vi "Finish.vi"   [LabVIEW 2017]
doc: "This VI is called just before exiting. It is expected to close I/O refnum, save collected data, etc."
types:
  T1 = typedef "WPI_JoystickDevRef.ctl" = cluster{"Device":T2}
  T2 = typedef "WPI_JoystickDeviceEnum.ctl" = enum16{"USB 0", "USB 1", "USB 2", "USB 3", "USB 4", "USB 5"}
  T3 = typedef "WPI_SolenoidDevRef.ctl" = cluster{"DevStatus":errorcluster, "Pneumatics Control Module":u8, "Forward Solenoid Channel":T4, "Reverse Solenoid Channel":T4}
  T4 = typedef "WPI_SolenoidChannel.ctl" = enum8{"Solenoid 0", "Solenoid 1", "Solenoid 2", "Solenoid 3", "Solenoid 4", "Solenoid 5", "Solenoid 6", "Solenoid 7", "Invalid"}
  T5 = typedef "WPI_EncoderDevRef.ctl" = cluster{"DevStatus":errorcluster, "EncoderIndex":T6, "CounterIndex":T7, "DistancePerCount":dbl, "Decoding Type":T8}
  T6 = typedef "FPGA_EncoderIdx.ctl" = enum8{"Enc 0", "Enc 1", "Enc 2", "Enc 3", "Enc 4", "Enc 5", "Enc 6", "Enc 7", "Invalid"}
  T7 = typedef "FPGA_CounterCtrSystemIndex.ctl" = enum8{"Ctr 0", "Ctr 1", "Ctr 2", "Ctr 3", "Ctr 4", "Ctr 5", "Ctr 6", "Ctr 7", "Invalid"}
  T8 = typedef "WPI_EncoderType.ctl" = enum16{"1x", "2x", "4x"}
  T9 = typedef "WPI_SwitchDevRef.ctl" = cluster{"DevStatus":errorcluster, "DIO Channel":T10, "CntIndex":T7, "Normally Closed":bool}
  T10 = typedef "FPGA_DIOChannel.ctl" = enum8{"DIO 0", "DIO 1", "DIO 2", "DIO 3", "DIO 4", "DIO 5", "DIO 6", "DIO 7", "DIO 8", "DIO 9", "DIO MXP 0", "DIO MXP 1", "DIO MXP 2", "DIO MXP 3", "DIO MXP 4", "DIO MXP 5", "DIO MXP 6", "DIO MXP 7", "DIO MXP 8", "DIO MXP 9", "DIO MXP 10", "DIO MXP 11", "DIO MXP 12", "DIO MXP 13", "DIO MXP 14", "DIO MXP 15", "SPI Port CS1", "SPI Port CS2", "SPI Port CS3", "SPI Port MISO", "SPI Port MOSI", "Invalid"}
  T11 = typedef "WPI_MotorControlDeviceRef.ctl" = cluster{"DeviceStatus":errorcluster, "Type":T12, "PWM":cluster{"PWM Channel":T13, "DeadBand":T14}, "CAN":cluster{"Device Number":u8, "SetOutput VI Ref":variant, "GetOutput VI Ref":variant, "Enable VI Ref":variant, "Disable VI Ref":variant, "Data":variant}, "Invert":bool, "DIO PWM":cluster{"PWM \"Enable\" Channel":T13, "DIOChannel":T10, "PWM Rate":dbl}}
  T12 = typedef "WPI_MotorControlType.ctl" = enum16{"PWM", "CAN", "DIO PWM"}
  T13 = typedef "FPGA_DIOPWMChannel.ctl" = enum8{"PWM 0", "PWM 1", "PWM 2", "PWM 3", "PWM 4", "PWM 5", "PWM 6", "PWM 7", "PWM 8", "PWM 9", "PWM MXP 0", "PWM MXP 1", "PWM MXP 2", "PWM MXP 3", "PWM MXP 4", "PWM MXP 5", "PWM MXP 6", "PWM MXP 7", "PWM MXP 8", "PWM MXP 9", "Invalid"}
  T14 = typedef "WPI_PWMDeadband.ctl" = cluster{"Name":string, "maxPositivePwm":i32, "minPositivePwm":i32, "centerPwm":i32, "maxNegativePwm":i32, "minNegativePwm":i32, "angularRange":u16}
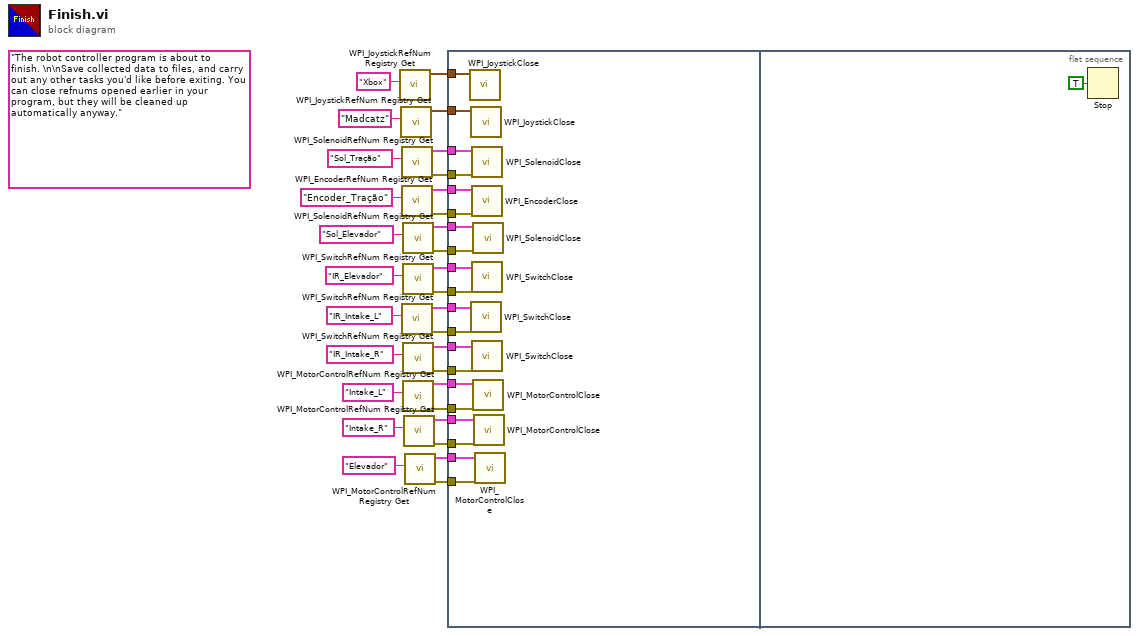
[diagram p0: block diagram]
diagram:
  (unwired) "The robot controller program is about to finish. \n\nSave collected data to files, and carry out any other tasks you'd like before exiting. You can close refnums opened earlier in your program, but they will be cleaned up automatically anyway."
  n1 = call <vilib>:"WPI_JoystickRefNum Registry Get.vi"("refnum name"="Xbox") -> ("JoystickDevRef"=w31:T1)  [unwired: 9 in, 1 out]
  n2 = call <vilib>:"WPI_JoystickRefNum Registry Get.vi"("refnum name"="Madcatz") -> ("JoystickDevRef"=w30:T1)  [unwired: 9 in, 1 out]
  n3 = call <vilib>:"WPI_SolenoidRefNum Registry Get.vi"("refnum name"="Sol_Tração") -> ("error out"=w26:errorcluster, "SolenoidDevRef"=w27:T3)  [unwired: 9 in]
  n4 = call <vilib>:"WPI_EncoderRefNum Registry Get.vi"("refnum name"="Encoder_Tração") -> ("error out"=w23:errorcluster, "EncoderDevRef"=w24:T5)  [unwired: 9 in]
  n5 = call <vilib>:"WPI_SwitchRefNum Registry Get.vi"("refnum name"="IR_Intake_L") -> ("error out"=w15:errorcluster, "SwitchDevRef"=w14:T9)  [unwired: 9 in]
  n6 = call <vilib>:"WPI_SolenoidRefNum Registry Get.vi"("refnum name"="Sol_Elevador") -> ("error out"=w21:errorcluster, "SolenoidDevRef"=w20:T3)  [unwired: 9 in]
  n7 = call <vilib>:"WPI_SwitchRefNum Registry Get.vi"("refnum name"="IR_Elevador") -> ("error out"=w17:errorcluster, "SwitchDevRef"=w18:T9)  [unwired: 9 in]
  n8 = call <vilib>:"WPI_SwitchRefNum Registry Get.vi"("refnum name"="IR_Intake_R") -> ("error out"=w12:errorcluster, "SwitchDevRef"=w13:T9)  [unwired: 9 in]
  n9 = call <vilib>:"WPI_MotorControlRefNum Registry Get.vi"("refnum name"="Intake_L") -> ("error out"=w8:errorcluster, "MotorControlDevRef"=w9:T11)  [unwired: 9 in]
  n10 = call <vilib>:"WPI_MotorControlRefNum Registry Get.vi"("refnum name"="Intake_R") -> ("error out"=w7:errorcluster, "MotorControlDevRef"=w6:T11)  [unwired: 9 in]
  n11 = call <vilib>:"WPI_MotorControlRefNum Registry Get.vi"("refnum name"="Elevador") -> ("error out"=w3:errorcluster, "MotorControlDevRef"=w2:T11)  [unwired: 9 in]
  n12 = flat-sequence {
    tunnel: w31 -> [w51]
    tunnel: w30 -> [w50]
    tunnel: w27 -> [w49]
    tunnel: w26 -> [w48]
    tunnel: w24 -> [w47]
    tunnel: w23 -> [w46]
    tunnel: w20 -> [w44]
    tunnel: w21 -> [w45]
    tunnel: w18 -> [w43]
    tunnel: w17 -> [w42]
    tunnel: w14 -> [w40]
    tunnel: w15 -> [w41]
    tunnel: w13 -> [w39]
    tunnel: w12 -> [w38]
    tunnel: w9 -> [w37]
    tunnel: w8 -> [w36]
    tunnel: w7 -> [w35]
    tunnel: w6 -> [w34]
    tunnel: w3 -> [w33]
    tunnel: w2 -> [w32]
    frame #0 {
      n13 = call <vilib>:"WPI_JoystickClose.vi"("JoystickDevRef"=w51) -> ()  [unwired: 11 in]
      n14 = call <vilib>:"WPI_JoystickClose.vi"("JoystickDevRef"=w50) -> ()  [unwired: 11 in]
      n15 = call <vilib>:"WPI_SwitchClose.vi"("error in (no error)"=w41, "SwitchDevRef"=w40) -> ()  [unwired: 9 in, 1 out]
      n16 = call <vilib>:"WPI_SolenoidClose.vi"("error in (no error)"=w48, "SolenoidDevRef"=w49) -> ()  [unwired: 9 in, 1 out]
      n17 = call <vilib>:"WPI_EncoderClose.vi"("error in (no error)"=w46, "EncoderDevRef"=w47) -> ()  [unwired: 9 in, 1 out]
      n18 = call <vilib>:"WPI_SwitchClose.vi"("error in (no error)"=w42, "SwitchDevRef"=w43) -> ()  [unwired: 9 in, 1 out]
      n19 = call <vilib>:"WPI_SwitchClose.vi"("error in (no error)"=w38, "SwitchDevRef"=w39) -> ()  [unwired: 9 in, 1 out]
      n20 = call <vilib>:"WPI_SolenoidClose.vi"("error in (no error)"=w45, "SolenoidDevRef"=w44) -> ()  [unwired: 9 in, 1 out]
      n21 = call <vilib>:"WPI_MotorControlClose.vi"("error in (no error)"=w36, "MotorControlDevRef"=w37) -> ()  [unwired: 9 in, 1 out]
      n22 = call <vilib>:"WPI_MotorControlClose.vi"("error in (no error)"=w35, "MotorControlDevRef"=w34) -> ()  [unwired: 9 in, 1 out]
      n23 = call <vilib>:"WPI_MotorControlClose.vi"("error in (no error)"=w33, "MotorControlDevRef"=w32) -> ()  [unwired: 9 in, 1 out]
    }
    frame #1 {
      n24 = Stop(stop? (T)=TRUE ("Quit")) -> ()
    }
  }
